vi "stop digital software pulse .vi"(11 "handle":u32) -> (2 "function return":bool, 3 "handle out":u32)   [LabVIEW 2020, in "cDaq.lvlib"]
doc: "DAQAPI bool stop_digital_software_pulse_(HDAQ handle);"
uses:
  cDaq.lvlib
  cDaq.dll
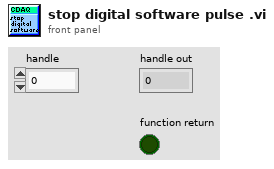
[diagram p1: front panel]
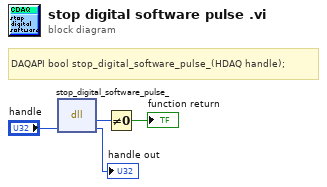
[diagram p0: block diagram]
diagram:
  # "DAQAPI bool stop_digital_software_pulse_(HDAQ handle);"
  n1 = dll-call lib="G:/CODE/01-Cplusplus/cDaq/doc/UsingWithLabview/cDaqlib/cDaq.*" fn="stop_digital_software_pulse_"("handle"="handle") -> (w3:u8, "handle"=→"handle out":u32)  [unwired: 3 in, 2 out]
  n2 = Not Equal To 0?(x=w3) -> (x != 0?=→"function return":bool)
